vi "Get Move Group Along An Arc Status.vi"(4 "error in (no error)":errorcluster, 6 "Group Number (1)":i32=1 min=1, 7 "VISA resource name":refnum<visa-resource-name>) -> (0 "error out":errorcluster, 2 "Arc  Parameters":T1 {"arc sweep angle (degrees)" format="%.6g"; "Second coordonate of arc center (units)" format="%.6g"; "first coordonate of arc center (units)" format="%.6g"}, 3 "VISA resource name out":refnum<visa-resource-name>)   [LabVIEW 2018, in "Newport ESP301.lvlib"]
doc: "this command reports the commanded center position of arc and sweep angle"
uses:
  Newport ESP301.lvlib
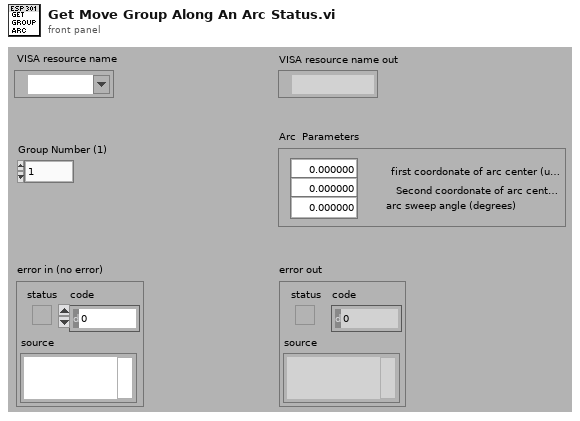
[diagram p1: front panel]
types:
  T1 = cluster{"first coordonate of arc center (units)":dbl, "Second coordonate of arc center (units)":dbl, "arc sweep angle (degrees)":dbl}
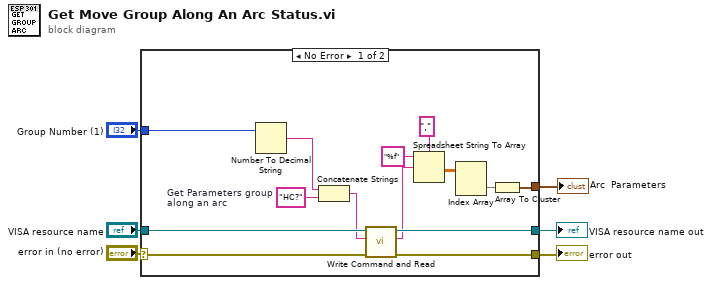
[diagram p0: block diagram]
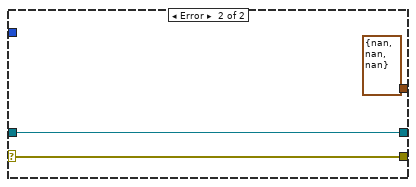
[diagram p2: hidden frame]
diagram:
  n1 = case shown="No Error" "error in (no error)" {
    selector: "error in (no error)" -> [w17 w23]
    tunnel: [w19 w23] -> w6
    tunnel: "VISA resource name" -> [w20 w22]
    tunnel: [w18 w22] -> w5
    tunnel: "Group Number (1)" -> [w13 _]
    tunnel: [w7 cluster{"[0]":dbl, "[1]":dbl, "[2]":dbl} {"[0]"=nan, "[1]"=nan, "[2]"=nan} ("cluster")] -> w1
    frame No Error {
      w16 = "HC?"  # Get Parameters group  along an arc
      n2 = Number To Decimal String(number=w13) -> (decimal integer string=w15:string)  [unwired: 1 in]
      n3 = Concatenate Strings(w15, w16) -> (w14:string)
      n4 = call "Write Command and Read.vi"("error in (no error)"=w17, "Command"=w14, "VISA resource name"=w20) -> ("error out"=w19:errorcluster, "Returned string"=w11:string, "VISA resource name out"=w18:refnum<visa-resource-name>)  [unwired: 4 in]
      n5 = Spreadsheet String To Array(delimiter (Tab)="," ("séparateur (Tabulation)"), format string="%f" ("chaîne de format"), spreadsheet string=w11) -> (array=w10:dbl[][])  [unwired: 1 in]
      n6 = Index Array(array=w10) -> (element=w9:dbl[])  [unwired: 2 in]
      n7 = Array To Cluster(array=w9) -> (cluster=w7:cluster{"[0]":dbl, "[1]":dbl, "[2]":dbl})
    }
    frame Error {
    }
  }
  "error out" <- w6
  "VISA resource name out" <- w5
  "Arc  Parameters" <- w1
